vi "lvstyx_get_dirent.vi"(2 "error in (no error)":errorcluster, 4 "index":i32, 5 "dir ptr":u32) -> (0 "error out":errorcluster, 1 "dirent ptr":u32)   [LabVIEW 2010, in "lib1299.lvlib"]
uses:
  lib1299.lvlib
  cstyx/win32/cstyx.dll
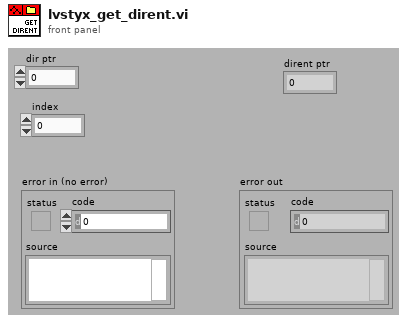
[diagram p1: front panel]
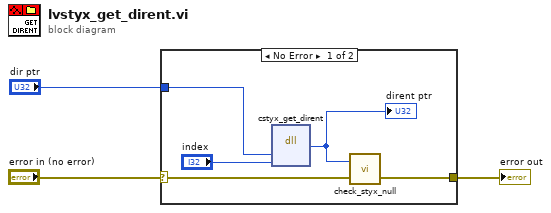
[diagram p0: block diagram]
diagram:
  n1 = case shown="No Error" "error in (no error)" {
    selector: "error in (no error)" -> [w7 w9]
    tunnel: "dir ptr" -> [w8 _]
    tunnel: [w6 w9] -> w2
    frame No Error {
      n2 = dll-call lib="C:/work/ads1299evm/lib_1299/Styx/cstyx/win32/cstyx.dll" fn="cstyx_get_dirent"("dir"=w8, "index"="index") -> ("dirent ptr"=w5:u32)  [unwired: 5 in, 2 out]
      "dirent ptr" <- w5
      n3 = call "check_styx_null.vi"("error in (no error)"=w7, "ptr"=w5) -> ("error out"=w6:errorcluster)  [unwired: 3 in]
    }
    frame Error {
    }
  }
  "error out" <- w2
